vi "Extension Attributes.vi"() -> ()   [LabVIEW 2024]
uses:
  <vilib>/Plug-In SDKs/Clients/Metadata/Extension.ctl
  <vilib>/Plug-In SDKs/Clients/Metadata/Hardware Item.ctl
  <vilib>/Plug-In SDKs/Clients/Data Store V1/Data Store Client.lvlibp/API/Data Store V1/Test Result.ctl
  <vilib>/Plug-In SDKs/Clients/Metadata/Outcome.ctl
  <vilib>/Plug-In SDKs/Clients/Metadata/Step.ctl
  <vilib>/Plug-In SDKs/Clients/Metadata Store V1/Metadata Store Client.lvlibp/API/Metadata Store V1/Register Schema (Path).vi
  <vilib>/Plug-In SDKs/Clients/Metadata Store V1/Metadata Store Client.lvlibp/API/Metadata Store V1/Create Hardware Item.vi
  <vilib>/Plug-In SDKs/Clients/Data Store V1/Data Store Client.lvlibp/API/Data Store V1/Publish Measurement (DBL Analog Waveform).vi
  <vilib>/Plug-In SDKs/Clients/Data Store V1/Data Store Client.lvlibp/API/Data Store V1/Read Data from Measurement (DBL Analog Waveform).vi
  <vilib>/Plug-In SDKs/Clients/Metadata Store V1/Metadata Store Client.lvlibp
  <vilib>/Plug-In SDKs/Clients/Metadata/NI Metadata Types.lvlib
  <vilib>/Plug-In SDKs/Clients/Data Store V1/Data Store Client.lvlibp
  <vilib>/measure/NI_MABase.lvlib
panel:
  out "queried data":waveform(dbl)(graph)
  out "measurement name":string
  out "hardware item ids":string[](array[string])
  out "log":string
  out "error out":errorcluster
  # "Extension Attributes\n\nIn this example:\n- Create metadata entities with extension attributes.\n- Publish waveform data with metadata attached.\n- Query the measurement based on extension attributes."
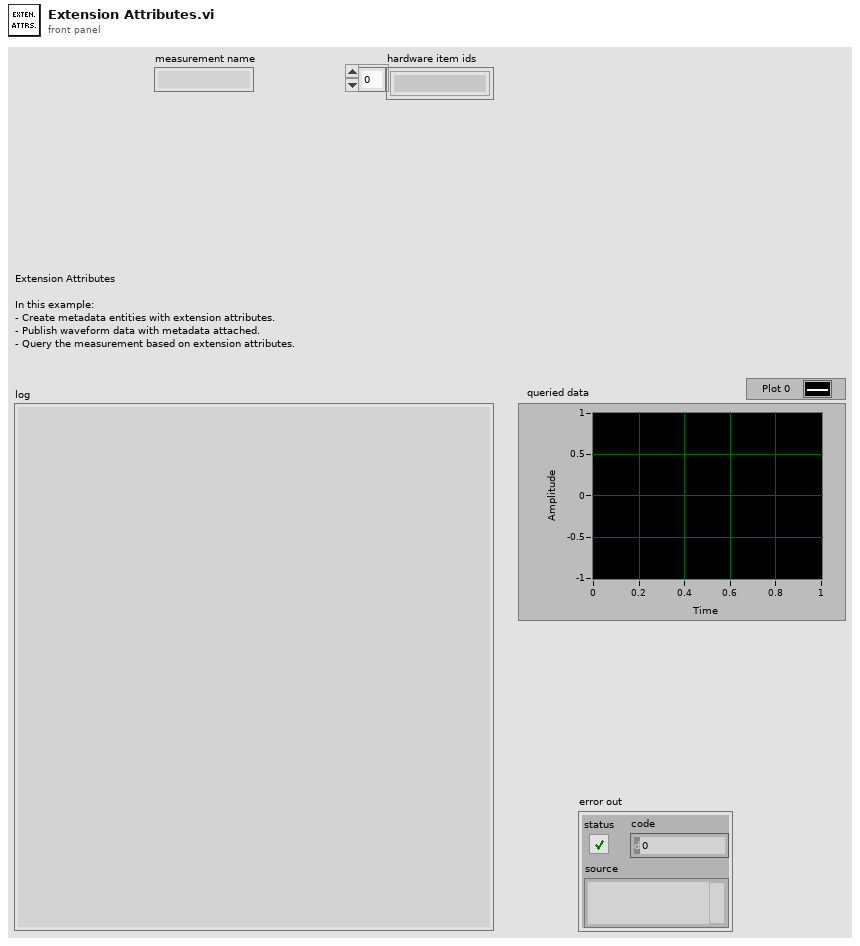
[diagram p1: front panel]
types:
  T1 = enum16{"Create Hardware Items With Extension Attributes", "Publish Measurement With Hardware", "Query Published Data"}
  T2 = typedef "NI Metadata Types.lvlib/Extension.ctl" = cluster{"name":string, "value":string}
  T3 = typedef "NI Metadata Types.lvlib/Hardware Item.ctl" = cluster{"model":string, "manufacturer":string, "part number":string, "serial number":string, "calibration due date":string, "asset identifier":string, "id":string, "link":string, "extensions":T2[], "schema id":string}
  T4 = typedef "NI Metadata Types.lvlib/Step.ctl" = cluster{"step name":string, "step type":string, "start date time":timestamp, "end date time":timestamp, "notes":string, "step id":string, "parent step id":string, "test result id":string, "test id":string, "link":string, "extensions":T2[], "schema id":string}
  T5 = typedef "Data Store Client.lvlibp/Test Result.ctl" = cluster{"test result name":string, "start date time":timestamp, "end date time":timestamp, "outcome":T6, "test result id":string, "uut instance id":string, "operator id":string, "test station id":string, "test description id":string, "software item ids":string[], "hardware item ids":string[], "test adapter ids":string[], "link":string, "extensions":T2[], "schema id":string}
  T6 = typedef "NI Metadata Types.lvlib/Outcome.ctl" = enum32{"Unspecified", "Passed", "Failed", "Indeterminate"}
  T7 = typedef "Data Store Client.lvlibp/Published Measurement.ctl" = cluster{"data moniker":T8, "published conditions":T9[], "published measurement id":string, "test result id":string, "step id":string, "software item ids":string[], "hardware item ids":string[], "test adapter ids":string[], "measurement name":string, "data type":string, "measurement notes":string, "start date time":timestamp, "end date time":timestamp, "outcome":T6, "parametric index":i32, "error information":T10}
  T8 = typedef "Data Store Client.lvlibp/Data Moniker.ctl" = cluster{"service location":string, "data source":string, "data instance":i64}
  T9 = typedef "Data Store Client.lvlibp/Published Condition.ctl" = cluster{"moniker":T8, "published condition id":string, "condition name":string, "condition type":string, "step id":string, "test result id":string}
  T10 = typedef "NI Metadata Types.lvlib/Error Information.ctl" = cluster{"error code":i32, "message":string, "source":string}
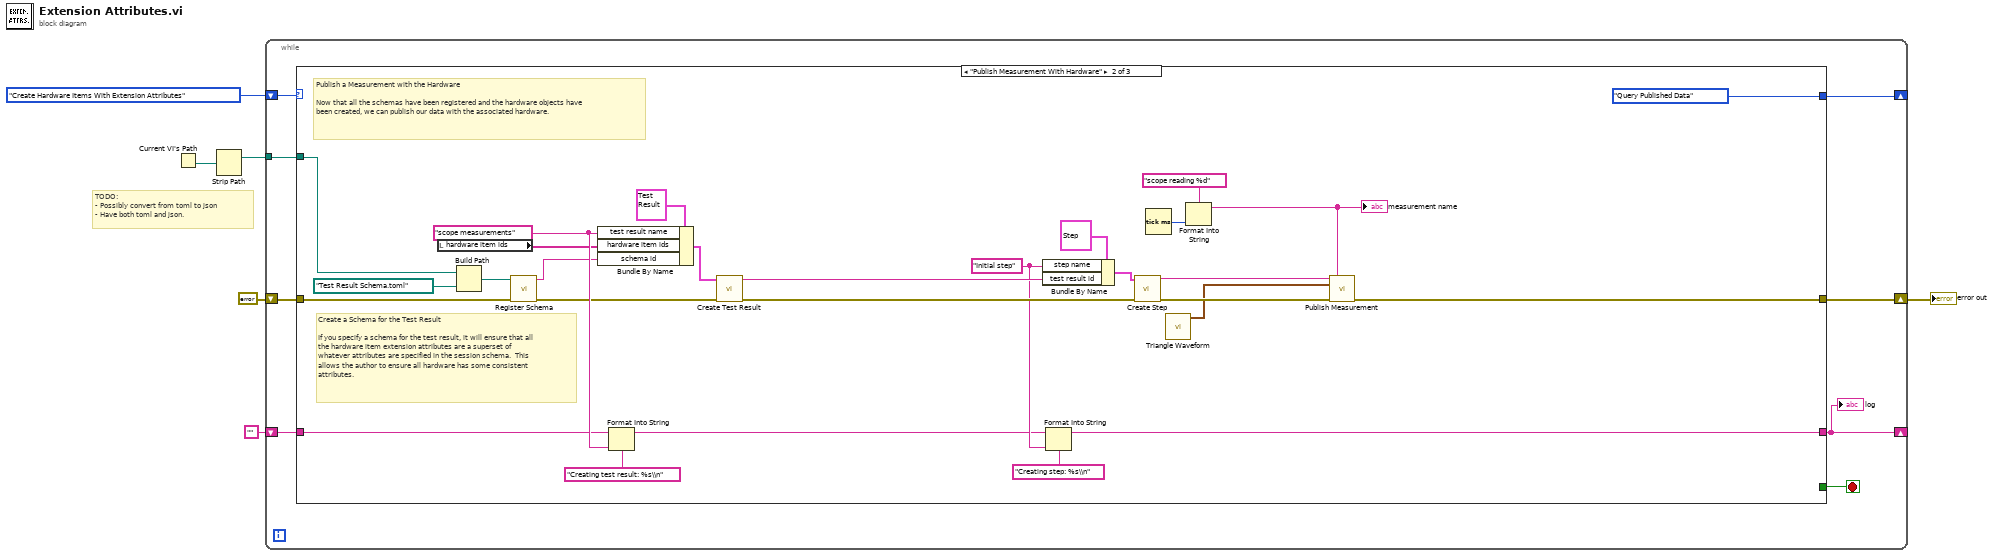
[diagram p0: block diagram]
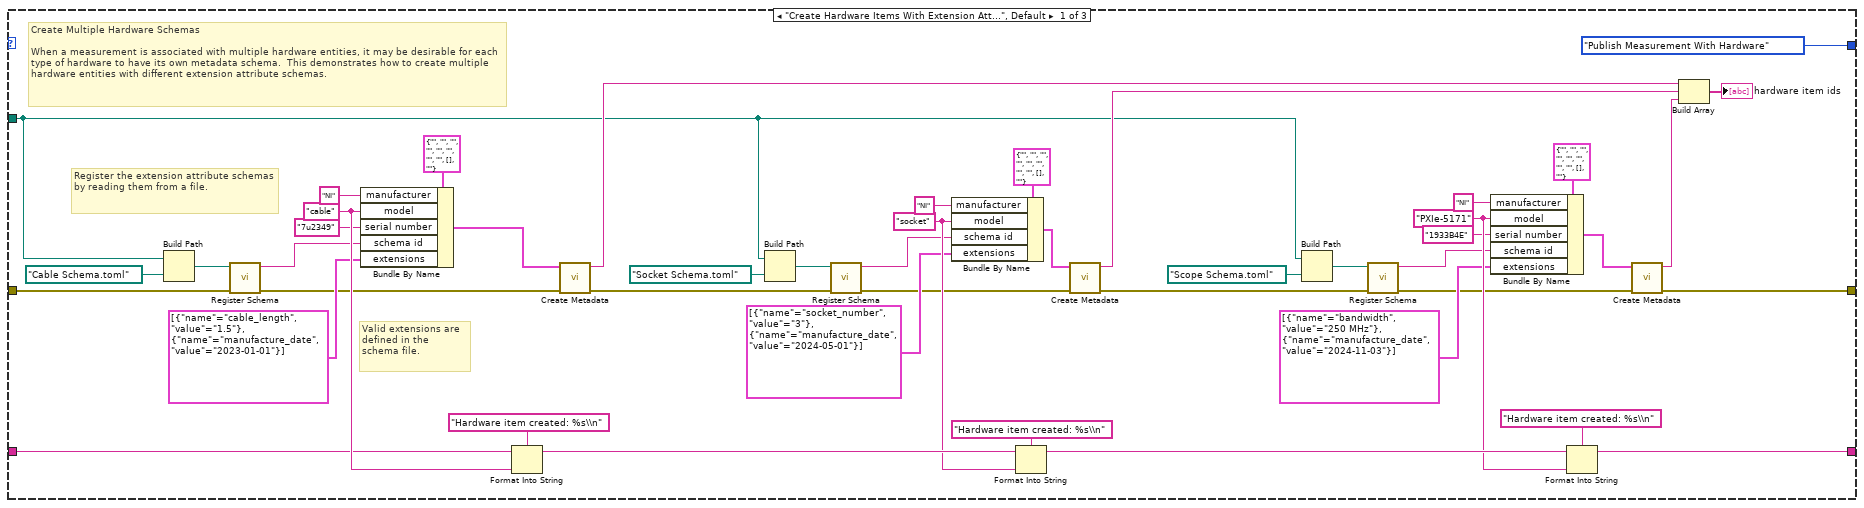
[diagram p2: hidden frame]
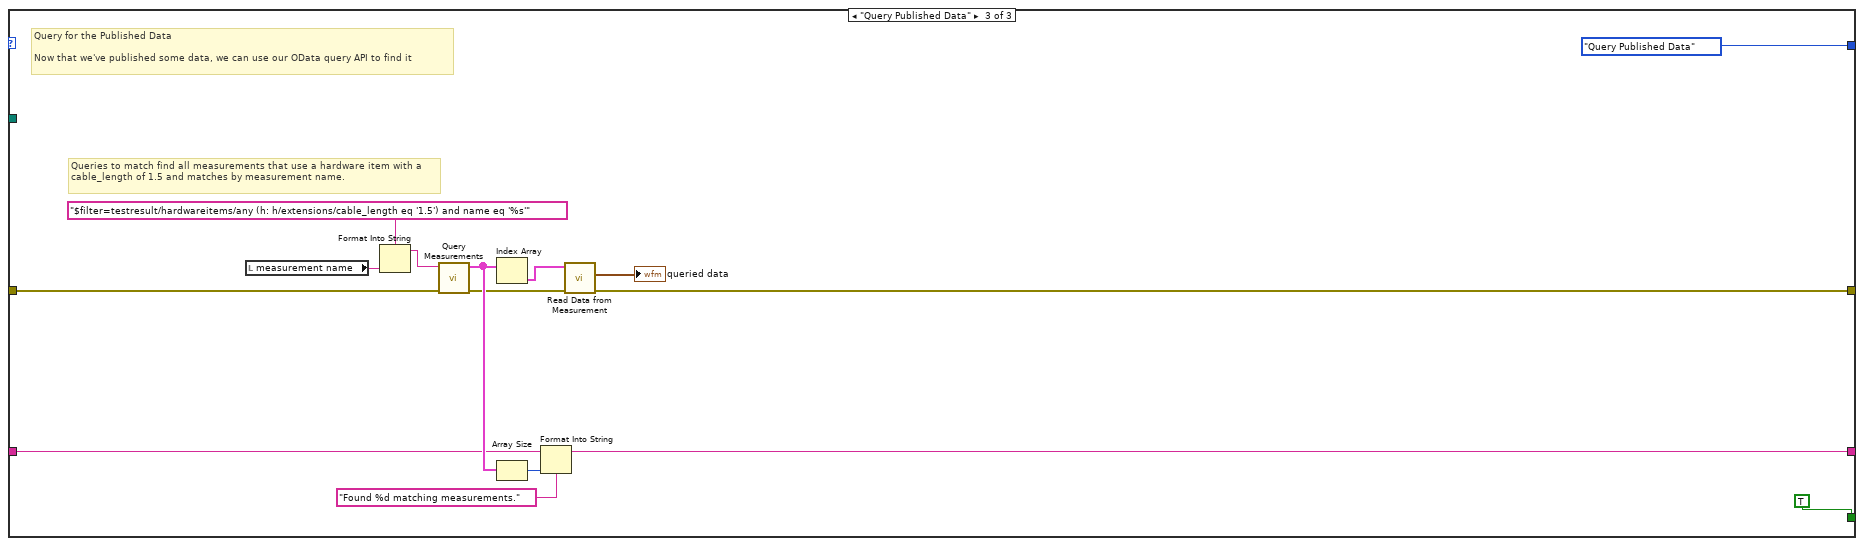
[diagram p3: hidden frame]
diagram:
  # "TODO:\n- Possibly convert from toml to json\n- Have both toml and json."
  n1 = Current VI's Path() -> (path=w2:path)
  n2 = Strip Path(path=w2) -> (stripped path=w1:path)  [unwired: 1 out]
  n3 = while {
    shift-right: [w13] -> w3
    shift-left: errorcluster {"status"=FALSE, "code"=0, "source"=""} ("error out") -> [w12]
    shift-right: [w10] -> _
    shift-left: "" -> [w11]
    shift-right: [w8] -> _
    shift-left: T1."Create Hardware Items With Extension Attributes" -> [w14]
    tunnel: w1 -> [w7]
    stop <- w9 stop-if-true
    n4 = case shown="\"Publish Measurement With Hardware\"" w14 {
      tunnel: [w60 w69 w95] -> w13
      tunnel: w12 -> [w29 w65 w98]
      tunnel: [w34 w68 w94] -> w10
      tunnel: w11 -> [w33 w70 w96]
      tunnel: [_ _ TRUE] -> w9
      tunnel: [T1."Publish Measurement With Hardware" T1."Query Published Data" T1."Query Published Data"] -> w8
      tunnel: w7 -> [w15 w61 _]
      frame "Create Hardware Items With Extension Attributes", Default {
        w57 = "PXIe-5171" ("model")
        w55 = "socket" ("socket model")
        w53 = "cable" ("model")
        # "Valid extensions are defined in the schema file."
        # "Create Multiple Hardware Schemas\n\nWhen a measurement is associated with multiple hardware entities, it may be desirable for each type of hardware to have its own metadata schema.  This demonstrates how to create multiple hardware entities with different extension attribute schemas."
        # "Register the extension attribute schemas by reading them from a file."
        n5 = Build Path(base path=w15, name or relative path=path "Cable Schema.toml" ("file (use dialog)")) -> (appended path=w27:path)
        n6 = call-poly <vilib>:"Register Schema.vi"("error in"=w29, "schema"=w27) -> ("error out"=w28:errorcluster, "schema id"=w26:string)  [unwired: 8 in]
        n7 = Bundle By Name(cluster=T3 {"model"="", "manufacturer"="", "part number"="", "serial number"="", "calibration due date"="", "asset identifier"="", "id"="", "link"="", "extensions"=[], "schema id"=""} ("hardware item"), "manufacturer"="NI", "model"=w53, "serial number"="7u2349", "schema id"=w26, "extensions"=T2[] [{"name"="cable_length", "value"="1.5"}, {"name"="manufacture_date", "value"="2023-01-01"}]) -> (w47:T3)
        n8 = Format Into String(format string="Hardware item created: %s\\n", initial string=w33, w53) -> (resulting string=w58:string)  [unwired: 1 in, 1 out]
        n9 = call-poly <vilib>:"Create Metadata.vi"("error in"=w28, "hardware item"=w47) -> ("error out"=w23:errorcluster, "hardware item id"=w40:string)  [unwired: 8 in]
        n10 = Build Path(base path=w15, name or relative path=path "Socket Schema.toml" ("file (use dialog)")) -> (appended path=w25:path)
        n11 = call-poly <vilib>:"Register Schema.vi"("error in"=w23, "schema"=w25) -> ("error out"=w24:errorcluster, "schema id"=w22:string)  [unwired: 8 in]
        n12 = Bundle By Name(cluster=T3 {"model"="", "manufacturer"="", "part number"="", "serial number"="", "calibration due date"="", "asset identifier"="", "id"="", "link"="", "extensions"=[], "schema id"=""} ("hardware item"), "manufacturer"="NI" ("socket manufacturer"), "model"=w55, "schema id"=w22, "extensions"=T2[] [{"name"="socket_number", "value"="3"}, {"name"="manufacture_date", "value"="2024-05-01"}] ("socket extensions")) -> (w45:T3)
        n13 = Format Into String(format string="Hardware item created: %s\\n", initial string=w58, w55) -> (resulting string=w59:string)  [unwired: 1 in, 1 out]
        n14 = call-poly <vilib>:"Create Metadata.vi"("error in"=w24, "hardware item"=w45) -> ("error out"=w18:errorcluster, "hardware item id"=w39:string)  [unwired: 8 in]
        n15 = Build Path(base path=w15, name or relative path=path "Scope Schema.toml" ("file (use dialog)")) -> (appended path=w20:path)
        n16 = call-poly <vilib>:"Register Schema.vi"("error in"=w18, "schema"=w20) -> ("error out"=w19:errorcluster, "schema id"=w17:string)  [unwired: 8 in]
        n17 = Bundle By Name(cluster=T3 {"model"="", "manufacturer"="", "part number"="", "serial number"="", "calibration due date"="", "asset identifier"="", "id"="", "link"="", "extensions"=[], "schema id"=""} ("scope"), "manufacturer"="NI", "model"=w57, "serial number"="1933B4E", "schema id"=w17, "extensions"=T2[] [{"name"="bandwidth", "value"="250 MHz"}, {"name"="manufacture_date", "value"="2024-11-03"}]) -> (w41:T3)
        n18 = Format Into String(format string="Hardware item created: %s\\n", initial string=w59, w57) -> (resulting string=w34:string)  [unwired: 1 in, 1 out]
        n19 = call-poly <vilib>:"Create Metadata.vi"("error in"=w19, "hardware item"=w41) -> ("error out"=w60:errorcluster, "hardware item id"=w38:string)  [unwired: 8 in]
        n20 = Build Array(w40, w39, w38) -> (→"hardware item ids":string[])
      }
      frame "Publish Measurement With Hardware" {
        w79 = "Initial step" ("step name")
        w86 = "scope measurements" ("test result name")
        # "Publish a Measurement with the Hardware\n\nNow that all the schemas have been registered and the hardware objects have been created, we can publish our data with the associated hardware."
        # "Create a Schema for the Test Result\n\nIf you specify a schema for the test result, it will ensure that all the hardware item extension attributes are a superset of whatever attributes are specified in the session schema.  This allows the author to ensure all hardware has some consistent attributes."
        n21 = local read "hardware item ids"() -> (w73:string[])
        n22 = Build Path(base path=w61, name or relative path=path "Test Result Schema.toml" ("file (use dialog)")) -> (appended path=w66:path)
        n23 = call-poly <vilib>:"Register Schema.vi"("error in"=w65, "schema"=w66) -> ("error out"=w64:errorcluster, "schema id"=w63:string)  [unwired: 8 in]
        n24 = Bundle By Name(cluster=T5 {"test result name"="", "start date time"=timestamp(0 s since 1904-01-01), "end date time"=timestamp(0 s since 1904-01-01), "outcome"=enum."Unspecified", "test result id"="", "uut instance id"="", "operator id"="", "test station id"="", "test description id"="", "software item ids"=[], "hardware item ids"=[], "test adapter ids"=[], "link"="", "extensions"=[], "schema id"=""} ("test result"), "test result name"=w86, "hardware item ids"=w73, "schema id"=w63) -> (w83:T5)
        n25 = Format Into String(format string="Creating test result: %s\\n", initial string=w70, w86) -> (resulting string=w72:string)  [unwired: 1 in, 1 out]
        n26 = call <vilib>:"Create Test Result.vi"("error in"=w64, "test result"=w83) -> ("error out"=w88:errorcluster, "test result id"=w87:string)  [unwired: 8 in]
        n27 = Bundle By Name(cluster=T4 {"step name"="", "step type"="", "start date time"=timestamp(0 s since 1904-01-01), "end date time"=timestamp(0 s since 1904-01-01), "notes"="", "step id"="", "parent step id"="", "test result id"="", "test id"="", "link"="", "extensions"=[], "schema id"=""} ("step"), "step name"=w79, "test result id"=w87) -> (w76:T4)
        n28 = Format Into String(format string="Creating step: %s\\n", initial string=w72, w79) -> (resulting string=w68:string)  [unwired: 1 in, 1 out]
        n29 = call <vilib>:"Create Step.vi"("error in"=w88, "step"=w76) -> ("error out"=w74:errorcluster, "step id"=w75:string)  [unwired: 8 in]
        n30 = Tick Count (ms)() -> (millisecond timer value=w81:u32)
        n31 = call <vilib>:"Triangle Waveform.vi"() -> ("signal out"=w71:waveform(dbl))  [unwired: 10 in, 1 out]
        n32 = Format Into String(format string="scope reading %d", w81) -> (resulting string=w82:string)  [unwired: 2 in, 1 out]
        "measurement name" <- w82
        n33 = call-poly <vilib>:"Publish Measurement.vi"("step id"=w75, "name"=w82, "waveform"=w71, "error in"=w74) -> ("error out"=w69:errorcluster)  [unwired: 9 in, 2 out]
      }
      frame "Query Published Data" {
        # "Queries to match find all measurements that use a hardware item with a cable_length of 1.5 and matches by measurement name."
        # "Query for the Published Data\n\nNow that we've published some data, we can use our OData query API to find it"
        n34 = local read "measurement name"() -> (w97:string)
        n35 = Format Into String(format string="$filter=testresult/hardwareitems/any (h: h/extensions/cable_length eq '1.5') and name eq '%s'" ("odata query"), w97) -> (resulting string=w90:string)  [unwired: 2 in, 1 out]
        n36 = call <vilib>:"Query Measurements.vi"("error in"=w98, "odata query"=w90) -> ("error out"=w99:errorcluster, "published measurements"=w101:T7[])  [unwired: 8 in]
        n37 = Index Array(array=w101) -> (element=w100:T7)  [unwired: 1 in]
        n38 = Array Size(array=w101) -> (size(s)=w103:i32)
        n39 = Format Into String(format string="Found %d matching measurements.", initial string=w96, w103) -> (resulting string=w94:string)  [unwired: 1 in, 1 out]
        n40 = call-poly <vilib>:"Read Data from Measurement.vi"("error in"=w99, "published measurement"=w100) -> ("error out"=w95:errorcluster, "waveform data"=→"queried data":waveform(dbl))  [unwired: 7 in, 1 out]
      }
    }
    "log" <- w10
  }
  "error out" <- w3
